vi "Keep Alive Interval.vi"(8 "error in (no error)":errorcluster, 9 "Connection Name":string, 11 "KeepAliveInterval (s)":i32) -> (0 "error out":errorcluster)   [LabVIEW 2018, in "LabSSH.lvlib"]
uses:
  LabSSH.lvlib
  FGV State..enum.ctl
  Z:/work/git/fpganow/MicroBlaze_lwIP/labview_fpga_nic/References/References/LabSSH.dll
  References/LabSSH.dll
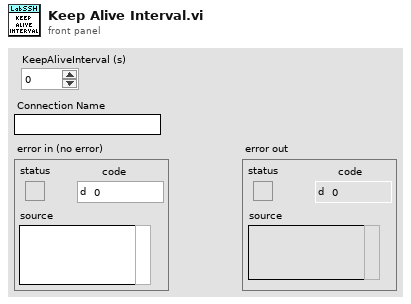
[diagram p1: front panel]
types:
  T1 = typedef "LabSSH.lvlib/FGV State..enum.ctl" = enum16{"GET", "SET"}
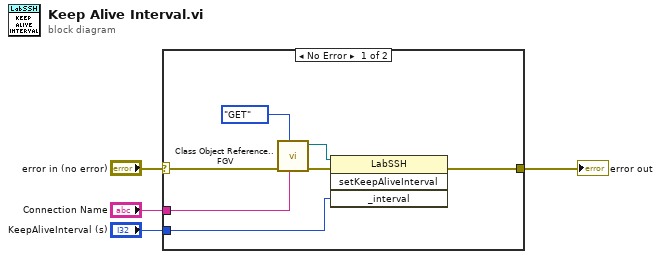
[diagram p0: block diagram]
diagram:
  n1 = case shown="No Error" "error in (no error)" {
    selector: "error in (no error)" -> [w8 w12]
    tunnel: [w7 w12] -> w3
    tunnel: "Connection Name" -> [w6 _]
    tunnel: "KeepAliveInterval (s)" -> [w5 _]
    frame No Error {
      n2 = call "Class Object Reference..FGV.vi"("Connection Name"=w6, "FGV State (GET)"=FGV_State..enum."GET" ("FGV State"), "error in (no error)"=w8) -> ("error out"=w9:errorcluster, "LabSSH ref out"=w10:refnum<k24>)  [unwired: 7 in]
      n3 = invoke on="Invoke Node" class="LabSSH" method="setKeepAliveInterval"(reference=w10, error in=w9, "_interval"=w5) -> (error out=w7:errorcluster)  [unwired: 1 in, 3 out]
    }
    frame Error {
    }
  }
  "error out" <- w3
